vi "Set Pump Phases Parameters(SubVI).vi"(0 "Send":bool, 1 "Pump resource in":refnum<visa-resource-name>, 3 "Pump error in":errorcluster, 5 "Valve Position":dbl, 7 "Pump direction":string, 9 "Units":string, 11 "Pump rate":dbl, 12 "Valve resource name in":refnum<visa-resource-name>, 14 "Valve error in":errorcluster) -> (4 "Pump resource name out":refnum<visa-resource-name>, 6 "pump error out":errorcluster, 10 "Valve resource name out":refnum<visa-resource-name>, 15 "Valve error out":errorcluster)   [LabVIEW 2020]
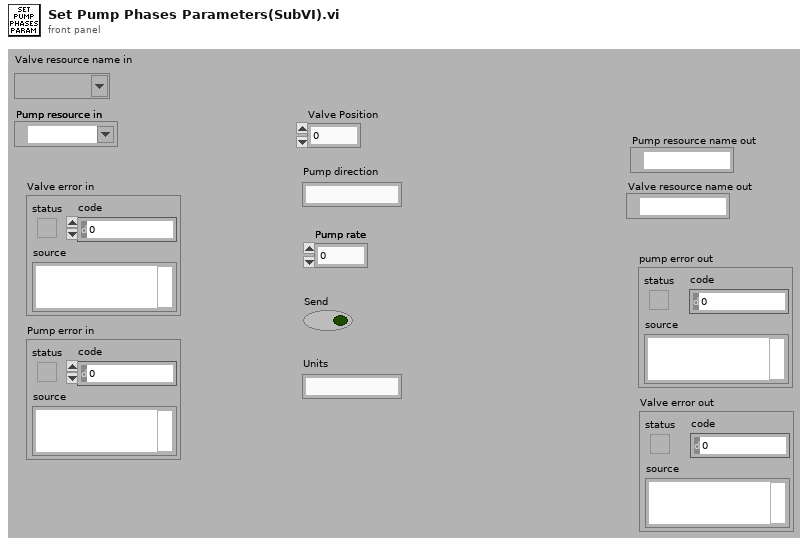
[diagram p1: front panel]
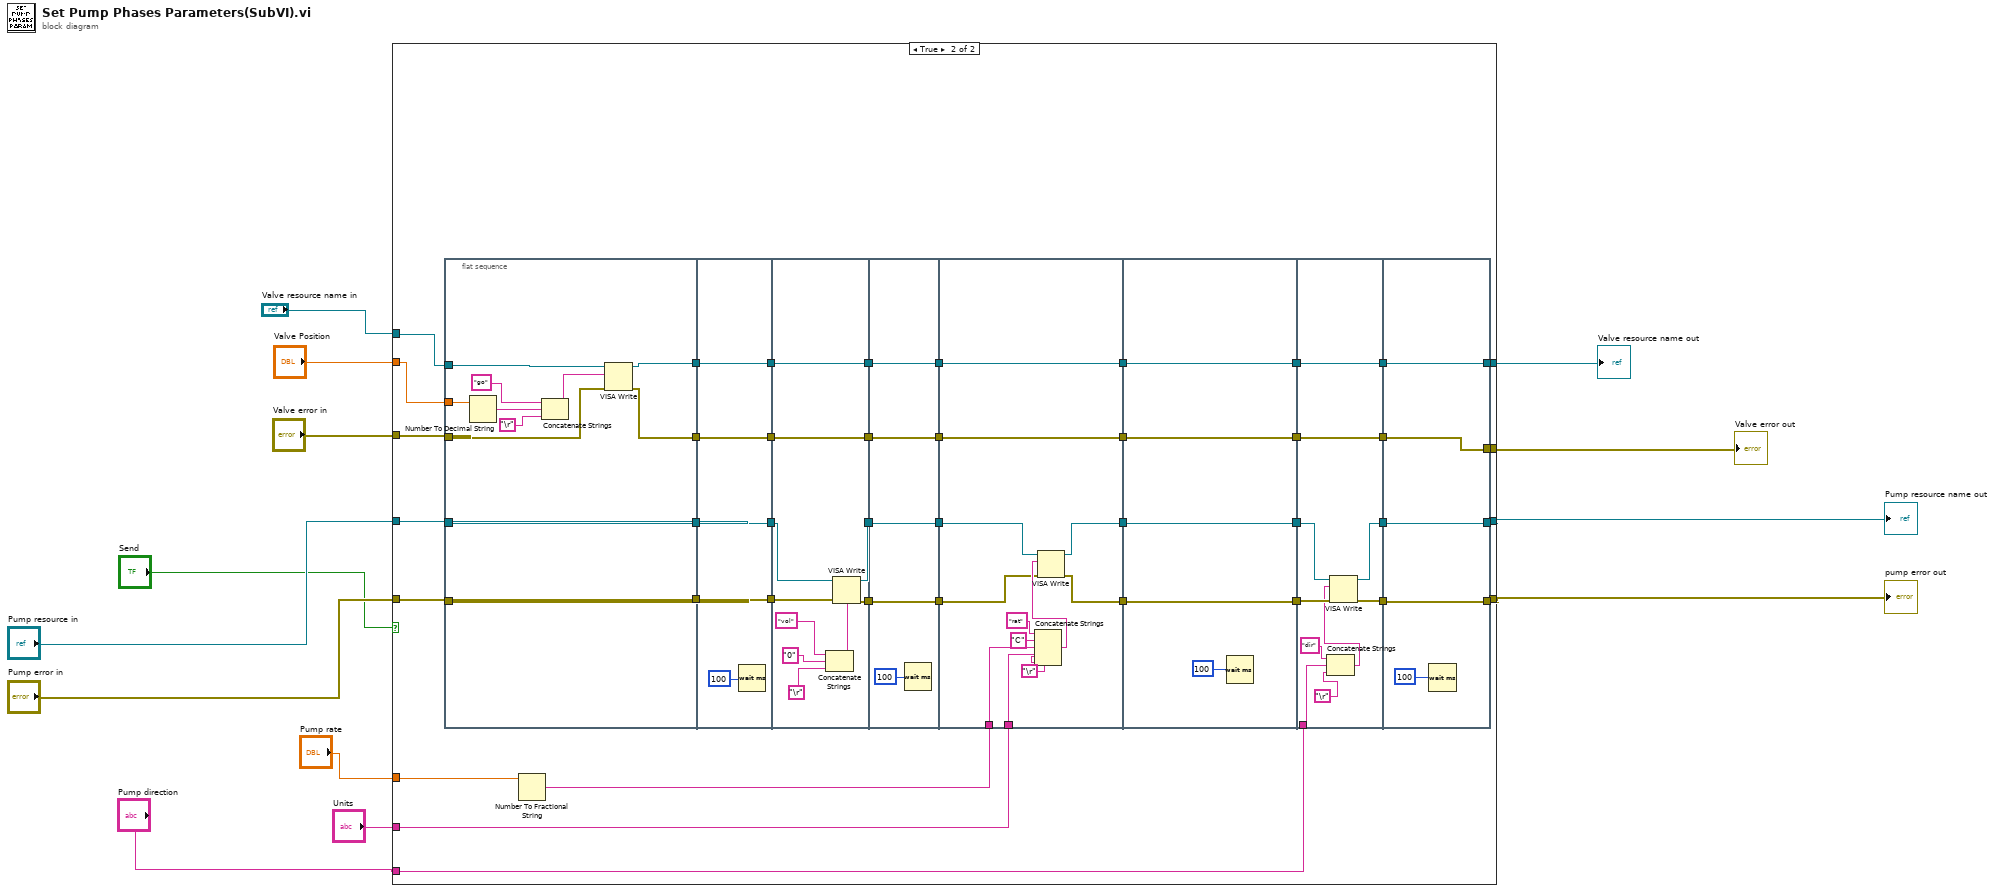
[diagram p0: block diagram]
diagram:
  n1 = case shown="True" "Send" {
    tunnel: "Pump resource in" -> [w17 w58]
    tunnel: "Pump error in" -> [w16 w57]
    tunnel: [w17 w56] -> w12
    tunnel: [w16 w55] -> w13
    tunnel: "Pump direction" -> [_ w52]
    tunnel: "Valve Position" -> [_ w48]
    tunnel: "Valve resource name in" -> [w15 w49]
    tunnel: "Valve error in" -> [w14 w47]
    tunnel: [w14 w38] -> w5
    tunnel: [w15 w33] -> w4
    tunnel: "Pump rate" -> [_ w20]
    tunnel: "Units" -> [_ w18]
    frame False {
    }
    frame True {
      n2 = flat-sequence {
        tunnel: w57 -> [w61]
        tunnel: w58 -> [w62]
        tunnel: w49 -> [w65]
        tunnel: w48 -> [w64]
        tunnel: w47 -> [w63]
        tunnel: [w62] -> w46
        tunnel: [w61] -> w44
        tunnel: [w60] -> w42
        tunnel: [w59] -> w37
        tunnel: w46 -> [w73]
        tunnel: [w73] -> w45
        tunnel: w44 -> [w72]
        tunnel: [w72] -> w43
        tunnel: w42 -> [w71]
        tunnel: [w71] -> w41
        tunnel: w37 -> [w70]
        tunnel: [w70] -> w36
        tunnel: [w83] -> w54
        tunnel: [w84] -> w53
        tunnel: w45 -> [w78]
        tunnel: w43 -> [w77]
        tunnel: w41 -> [w76]
        tunnel: [w76] -> w40
        tunnel: w36 -> [w75]
        tunnel: [w75] -> w35
        tunnel: w54 -> [w89]
        tunnel: w53 -> [w88]
        tunnel: [w89] -> w28
        tunnel: [w88] -> w26
        tunnel: w40 -> [w86]
        tunnel: [w86] -> w24
        tunnel: w35 -> [w85]
        tunnel: [w85] -> w22
        tunnel: w28 -> [w96]
        tunnel: [w94] -> w27
        tunnel: w26 -> [w95]
        tunnel: [w93] -> w25
        tunnel: w24 -> [w101]
        tunnel: [w101] -> w23
        tunnel: w22 -> [w100]
        tunnel: [w100] -> w21
        tunnel: w19 -> [w92]
        tunnel: w18 -> [w91]
        tunnel: w27 -> [w106]
        tunnel: [w106] -> w32
        tunnel: w25 -> [w105]
        tunnel: [w105] -> w31
        tunnel: w23 -> [w104]
        tunnel: [w104] -> w30
        tunnel: w21 -> [w103]
        tunnel: [w103] -> w29
        tunnel: w32 -> [w116]
        tunnel: w31 -> [w113]
        tunnel: w52 -> [w109]
        tunnel: [w115] -> w51
        tunnel: [w114] -> w50
        tunnel: w30 -> [w108]
        tunnel: [w108] -> w39
        tunnel: w29 -> [w107]
        tunnel: [w107] -> w34
        tunnel: [w120] -> w55
        tunnel: [w121] -> w56
        tunnel: w51 -> [w121]
        tunnel: w50 -> [w120]
        tunnel: w39 -> [w118]
        tunnel: [w118] -> w38
        tunnel: w34 -> [w117]
        tunnel: [w117] -> w33
        frame #0 {
          n3 = Number To Decimal String(number=w64) -> (decimal integer string=w69:string)  [unwired: 1 in]
          n4 = Concatenate Strings("go", w69, "\r") -> (w68:string)
          n5 = VISA Write(VISA resource name=w65, write buffer=w68, error in (no error)=w63) -> (VISA resource name out=w59:refnum<visa-resource-name>, error out=w60:errorcluster)  [unwired: 1 out]
        }
        frame #1 {
          n6 = Wait (ms)(milliseconds to wait=u32 100) -> ()  [unwired: 1 out]
        }
        frame #2 {
          n7 = Concatenate Strings("vol" ("string"), "0" ("string"), "\r") -> (w80:string)
          n8 = VISA Write(VISA resource name=w78, write buffer=w80, error in (no error)=w77) -> (VISA resource name out=w83:refnum<visa-resource-name>, error out=w84:errorcluster)  [unwired: 1 out]
        }
        frame #3 {
          n9 = Wait (ms)(milliseconds to wait=u32 100) -> ()  [unwired: 1 out]
        }
        frame #4 {
          n10 = Concatenate Strings("rat" ("string"), "C" ("string"), w92, w91, "\r") -> (w99:string)
          n11 = VISA Write(VISA resource name=w96, write buffer=w99, error in (no error)=w95) -> (VISA resource name out=w94:refnum<visa-resource-name>, error out=w93:errorcluster)  [unwired: 1 out]
        }
        frame #5 {
          n12 = Wait (ms)(milliseconds to wait=u32 100) -> ()  [unwired: 1 out]
        }
        frame #6 {
          n13 = Concatenate Strings("dir" ("string"), w109, "\r") -> (w112:string)
          n14 = VISA Write(VISA resource name=w116, write buffer=w112, error in (no error)=w113) -> (VISA resource name out=w115:refnum<visa-resource-name>, error out=w114:errorcluster)  [unwired: 1 out]
        }
        frame #7 {
          n15 = Wait (ms)(milliseconds to wait=u32 100) -> ()  [unwired: 1 out]
        }
      }
      n16 = Number To Fractional String(number=w20) -> (F-format string=w19:string)  [unwired: 3 in]
    }
  }
  "pump error out" <- w13
  "Pump resource name out" <- w12
  "Valve error out" <- w5
  "Valve resource name out" <- w4
